vi "SM DEMO.vi"() -> ()   [LabVIEW 2022 SP3, in "StateMachine.lvlib" / "HSE-State-Machine.lvlib"]
doc: "Demonstrates the use of the HSE-State Machine and can be used as a Copy and Paste Template.\n\n____\nHAMPEL SOFTWARE ENGINEERING v2.6.0 (2023-12-19 10:54)"
uses:
  HSE-State-Machine.lvlib
  SM_States.ctl
  SM_Transitions.ctl
  <vilib>/Delacor/Delacor QMH/Libraries/Message Queue_class/Delacor_lib_QMH_Message Queue.lvclass
  <vilib>/Hampel Software Engineering/HSE Logger/hse-logger.lvlib
  Libraries/hse-libraries/Source/hse-dqmh/hse-dqmh.lvlib
panel:
  in  "stop":bool
  in  "Transition":T1=enum."Initialization finished"
  out "SM Exception":errorcluster
  in  "Polling Loop Signal":bool
  out "DEMO State":T2
  # "When HSE-State-Machine.lvlib is copied to another Module\nthan HSE State-Machine-Singleton.lvlib\nright click on the lvlib and select Remove From Library"
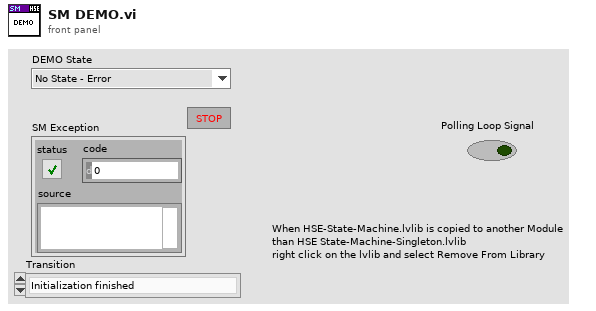
[diagram p1: front panel]
types:
  T1 = typedef "StateMachine.lvlib/HSE-State-Machine.lvlib/SM_Transitions.ctl" = enum16{"No Transition", "Exception", "Reset", "Initialization finished", "Process started", "Trigger detected", "Exit"}
  T2 = typedef "StateMachine.lvlib/HSE-State-Machine.lvlib/SM_States.ctl" = enum16{"No State - Error", "Error - Waiting For Action", "Initialising", "Standing by (idle)", "Waiting for External Trigger", "Polling for Signal Change", "Exiting"}
  T3 = typedef "StateMachine.lvlib/HSE-State-Machine.lvlib/SM Polling Actions--enum.ctl" = enum16{"Check transitions...", "Leave this state!"}
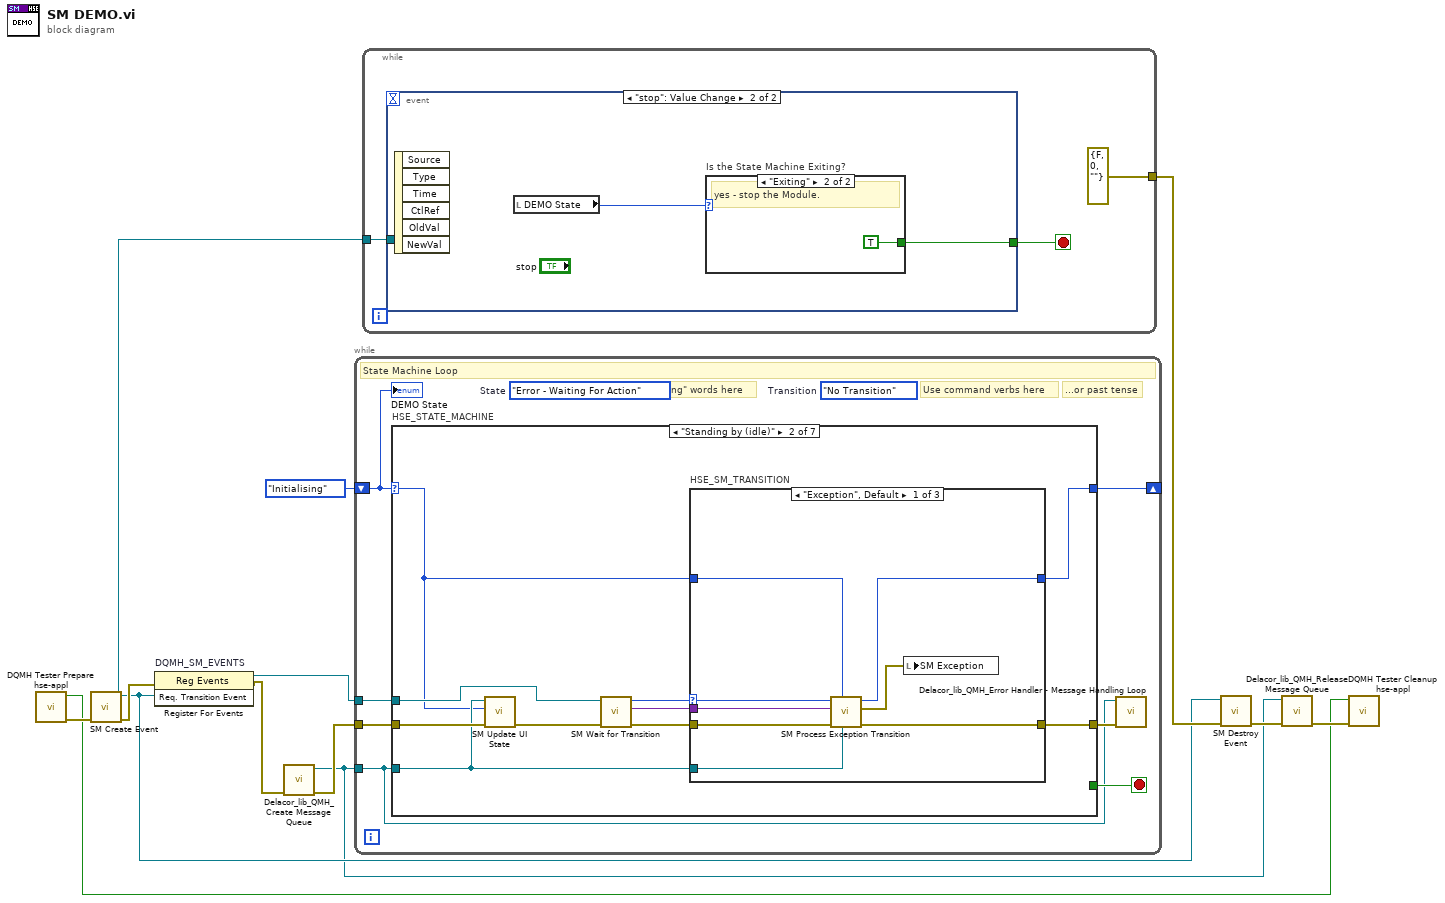
[diagram p0: block diagram]
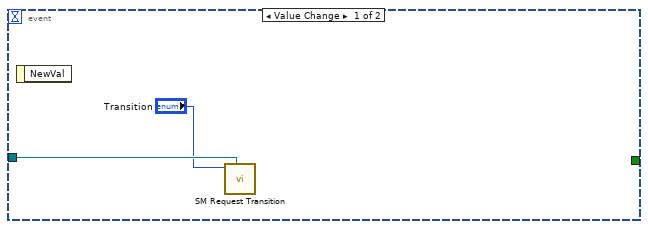
[diagram p2: hidden frame]
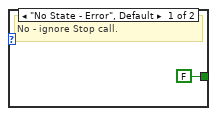
[diagram p3: hidden frame]
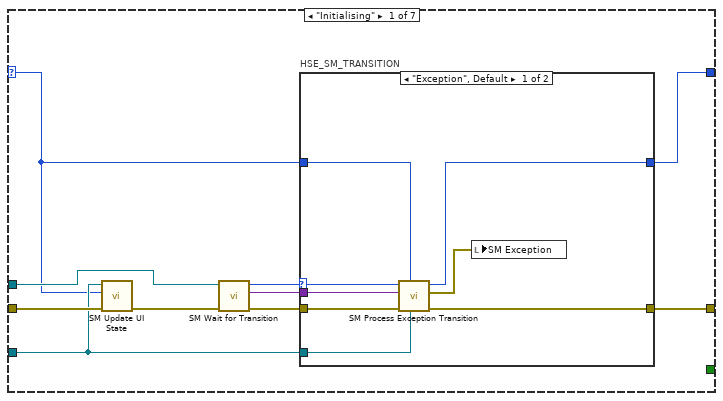
[diagram p4: hidden frame]
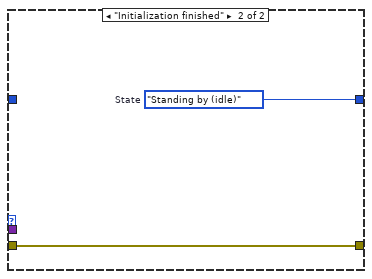
[diagram p5: hidden frame]
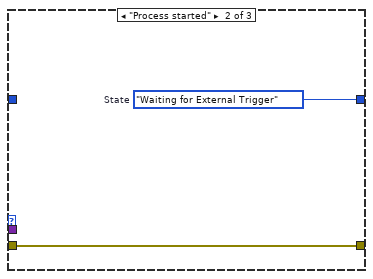
[diagram p6: hidden frame]
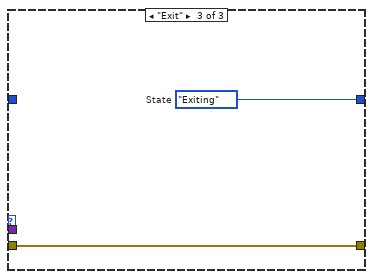
[diagram p7: hidden frame]
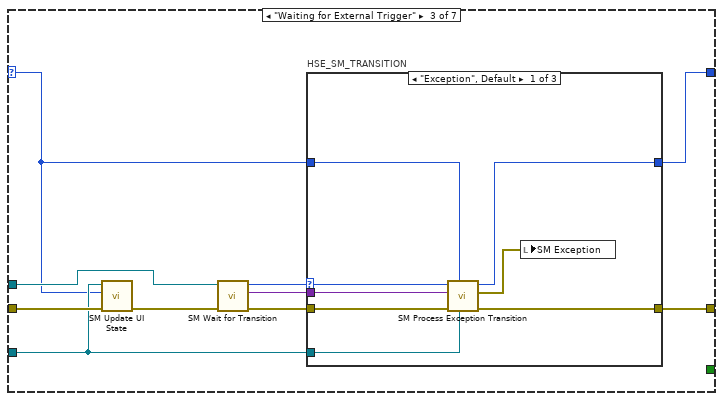
[diagram p8: hidden frame]
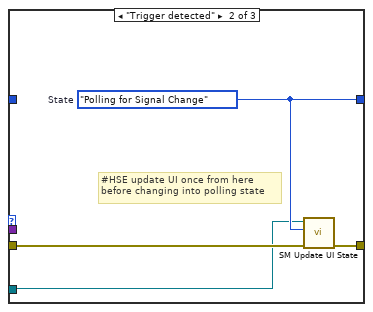
[diagram p9: hidden frame]
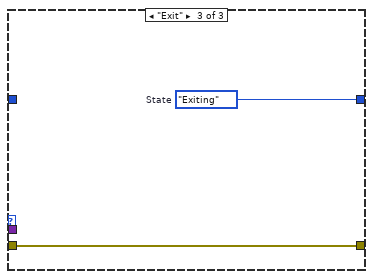
[diagram p10: hidden frame]
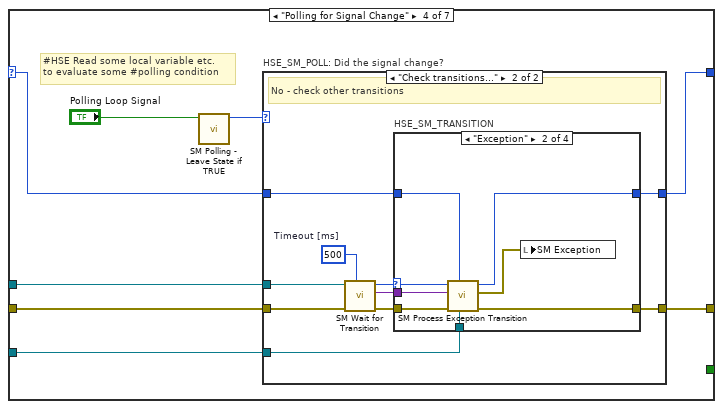
[diagram p11: hidden frame]
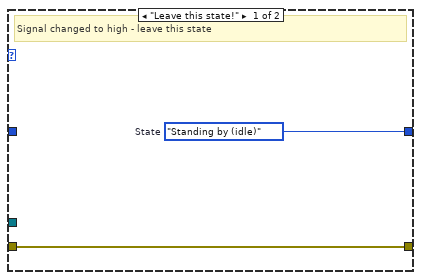
[diagram p12: hidden frame]
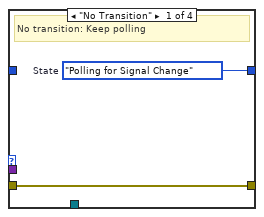
[diagram p13: hidden frame]
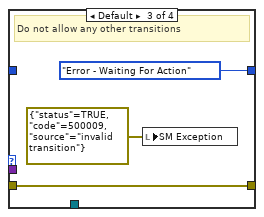
[diagram p14: hidden frame]
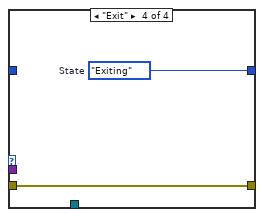
[diagram p15: hidden frame]
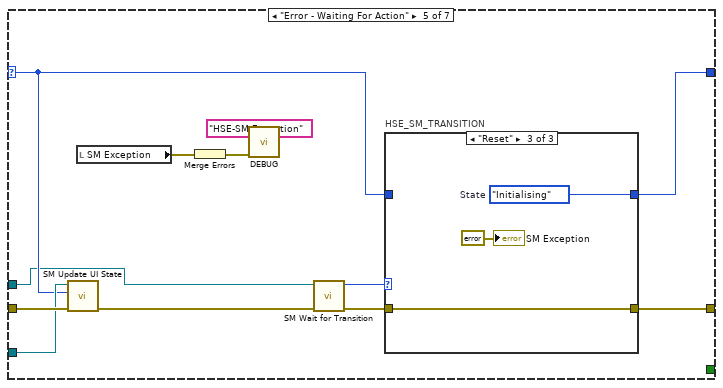
[diagram p16: hidden frame]
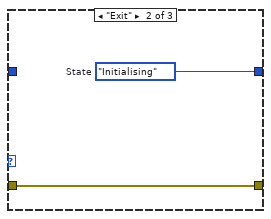
[diagram p18: hidden frame]
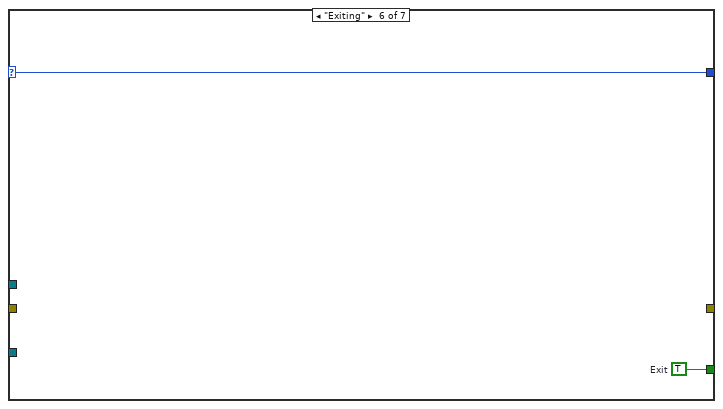
[diagram p19: hidden frame]
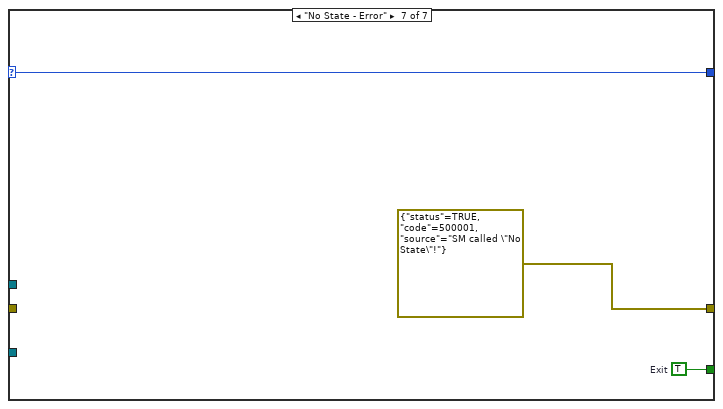
[diagram p20: hidden frame]
diagram:
  n1 = call "DQMH Tester Prepare hse-appl.vi"() -> ("error out"=w2:errorcluster, "Started?"=w1:bool)  [unwired: 8 in, 2 out]
  n2 = call "SM Create Event.vi"("error in (no error)"=w2) -> ("error out"=w10:errorcluster, "Req. Transition Event"=w8:refnum<user-event>)  [unwired: 9 in]
  n3 = register-events "DQMH_SM_EVENTS"(error in=w10, w8) -> (reference out=w9:refnum<event-registration>, error out=w6:errorcluster)  [unwired: 1 in]
  n4 = call <vilib>:"Delacor_lib_QMH_Create Message Queue.vi"("error in"=w6) -> ("error out"=w12:errorcluster, "Message Queue"=w4:refnum<class "Delacor_lib_QMH_Message Queue.lvclass">)  [unwired: 9 in]
  n5 = while {
    shift-right: [w18] -> _
    shift-left: SM_States."Initialising" ("State") -> [w19]
    tunnel: w4 -> [w13]
    tunnel: w9 -> [w15]
    tunnel: w12 -> [w14]
    stop <- w17 stop-if-true
    (unwired) SM_States."Error - Waiting For Action"  # State
    (unwired) SM_Transitions."No Transition"  # Transition
    # "...or past tense"
    # "Use command verbs here"
    # "Use \"-ing\" words here"
    # "State Machine Loop"
    n6 = case "HSE_STATE_MACHINE" shown="\"Standing by (idle)\"" w19 {
      selector: w19 -> [w20 w40 w62 w86 w122 w141 w144]
      tunnel: [w25 w45 w67 w92 w123 w141 w144] -> w18
      tunnel: [_ _ _ _ _ w140 w143] -> w17
      tunnel: w13 -> [w21 w41 w63 w90 w131 _ _]
      tunnel: [w24 w44 w66 w91 w125 _ errorcluster {"status"=TRUE, "code"=500001, "source"="SM called \"No State\"!"} ("error out")] -> w16
      tunnel: w15 -> [w22 w42 w64 w89 w121 _ _]
      tunnel: w14 -> [w29 w49 w71 w93 w132 _ _]
      frame "Initialising" {
        n7 = call "SM Update UI State.vi"("error in (no error)"=w29, "State"=w20, "Message Queue In"=w21) -> ("error out"=w23:errorcluster)  [unwired: 7 in, 1 out]
        n8 = call "SM Wait for Transition.vi"("error in (no error)"=w23, "Event Registration Refnum"=w22) -> ("error out"=w27:errorcluster, "Data"=w26:variant, "Transition"=w28:T1)  [unwired: 7 in]
        n9 = case "HSE_SM_TRANSITION" shown="\"Exception\", Default" w28 {
          selector: w28 -> [w30 _]
          tunnel: w27 -> [w37 w39]
          tunnel: w26 -> [w36 _]
          tunnel: [w32 w38] -> w25
          tunnel: [w35 w39] -> w24
          tunnel: w21 -> [w33 _]
          tunnel: w20 -> [w31 _]
          frame "Exception", Default {
            n10 = call "SM Process Exception Transition.vi"("Message Queue In"=w33, "Exception State"=w31, "error in (no error)"=w37, "Data"=w36, "Exception Transition"=w30) -> ("error out"=w35:errorcluster, "Exception"=w34:errorcluster, "State"=w32:T2)  [unwired: 4 in]
            n11 = local write "SM Exception"(w34) -> ()
          }
          frame "Initialization finished" {
            w38 = SM_States."Standing by (idle)"  # State
          }
        }
      }
      frame "Standing by (idle)" {
        n12 = call "SM Update UI State.vi"("error in (no error)"=w49, "State"=w40, "Message Queue In"=w41) -> ("error out"=w43:errorcluster)  [unwired: 7 in, 1 out]
        n13 = call "SM Wait for Transition.vi"("error in (no error)"=w43, "Event Registration Refnum"=w42) -> ("error out"=w47:errorcluster, "Data"=w46:variant, "Transition"=w48:T1)  [unwired: 7 in]
        n14 = case "HSE_SM_TRANSITION" shown="\"Exception\", Default" w48 {
          selector: w48 -> [w52 _ _]
          tunnel: w47 -> [w57 w59 w61]
          tunnel: w46 -> [w56 _ _]
          tunnel: [w51 w58 w60] -> w45
          tunnel: [w55 w59 w61] -> w44
          tunnel: w41 -> [w53 _ _]
          tunnel: w40 -> [w50 _ _]
          frame "Exception", Default {
            n15 = call "SM Process Exception Transition.vi"("Message Queue In"=w53, "Exception State"=w50, "error in (no error)"=w57, "Data"=w56, "Exception Transition"=w52) -> ("error out"=w55:errorcluster, "Exception"=w54:errorcluster, "State"=w51:T2)  [unwired: 4 in]
            n16 = local write "SM Exception"(w54) -> ()
          }
          frame "Process started" {
            w58 = SM_States."Waiting for External Trigger"  # State
          }
          frame "Exit" {
            w60 = SM_States."Exiting"  # State
          }
        }
      }
      frame "Waiting for External Trigger" {
        n17 = call "SM Update UI State.vi"("error in (no error)"=w71, "State"=w62, "Message Queue In"=w63) -> ("error out"=w65:errorcluster)  [unwired: 7 in, 1 out]
        n18 = call "SM Wait for Transition.vi"("error in (no error)"=w65, "Event Registration Refnum"=w64) -> ("error out"=w69:errorcluster, "Data"=w68:variant, "Transition"=w70:T1)  [unwired: 7 in]
        n19 = case "HSE_SM_TRANSITION" shown="\"Exception\", Default" w70 {
          selector: w70 -> [w72 _ _]
          tunnel: w69 -> [w79 w83 w85]
          tunnel: w68 -> [w78 _ _]
          tunnel: [w74 w81 w84] -> w67
          tunnel: [w77 w82 w85] -> w66
          tunnel: w63 -> [w75 w80 _]
          tunnel: w62 -> [w73 _ _]
          frame "Exception", Default {
            n20 = call "SM Process Exception Transition.vi"("Message Queue In"=w75, "Exception State"=w73, "error in (no error)"=w79, "Data"=w78, "Exception Transition"=w72) -> ("error out"=w77:errorcluster, "Exception"=w76:errorcluster, "State"=w74:T2)  [unwired: 4 in]
            n21 = local write "SM Exception"(w76) -> ()
          }
          frame "Trigger detected" {
            w81 = SM_States."Polling for Signal Change"  # State
            # "#HSE update UI once from here\nbefore changing into polling state"
            n22 = call "SM Update UI State.vi"("error in (no error)"=w83, "State"=w81, "Message Queue In"=w80) -> ("error out"=w82:errorcluster)  [unwired: 7 in, 1 out]
          }
          frame "Exit" {
            w84 = SM_States."Exiting"  # State
          }
        }
      }
      frame "Polling for Signal Change" {
        # "#HSE Read some local variable etc. \nto evaluate some #polling condition"
        n23 = call "SM Polling - Leave State if TRUE.vi"("Boolean Condition"="Polling Loop Signal") -> ("Polling Action"=w88:T3)  [unwired: 10 in]
        n24 = case "HSE_SM_POLL: Did the signal change?" shown="\"Check transitions...\"" w88 {
          tunnel: w93 -> [w94 w105]
          tunnel: [w95 w101] -> w92
          tunnel: [w94 w100] -> w91
          tunnel: w90 -> [_ w99]
          tunnel: w89 -> [_ w98]
          tunnel: w86 -> [_ w96]
          frame "Leave this state!" {
            w95 = SM_States."Standing by (idle)"  # State
            # "Signal changed to high - leave this state"
          }
          frame "Check transitions..." {
            w97 = 500  # Timeout [ms]
            # "No - check other transitions"
            n25 = call "SM Wait for Transition.vi"("Timeout [ms]"=w97, "error in (no error)"=w105, "Event Registration Refnum"=w98) -> ("error out"=w103:errorcluster, "Data"=w102:variant, "Transition"=w104:T1)  [unwired: 6 in]
            n26 = case "HSE_SM_TRANSITION" shown="\"Exception\"" w104 {
              selector: w104 -> [_ w110 _ _]
              tunnel: w103 -> [w106 w115 w117 w120]
              tunnel: w102 -> [_ w114 _ _]
              tunnel: [w107 w109 SM_States."Error - Waiting For Action" ("State") w119] -> w101
              tunnel: [w106 w113 w117 w120] -> w100
              tunnel: w99 -> [_ w111 _ _]
              tunnel: w96 -> [_ w108 _ _]
              frame "No Transition" {
                w107 = SM_States."Polling for Signal Change"  # State
                # "No transition: Keep polling"
              }
              frame "Exception" {
                n27 = call "SM Process Exception Transition.vi"("Message Queue In"=w111, "Exception State"=w108, "error in (no error)"=w115, "Data"=w114, "Exception Transition"=w110) -> ("error out"=w113:errorcluster, "Exception"=w112:errorcluster, "State"=w109:T2)  [unwired: 4 in]
                n28 = local write "SM Exception"(w112) -> ()
              }
              frame Default {
                # "Do not allow any other transitions"
                n29 = local write "SM Exception"(errorcluster {"status"=TRUE, "code"=500009, "source"="invalid transition"} ("SM Exception")) -> ()
              }
              frame "Exit" {
                w119 = SM_States."Exiting"  # State
              }
            }
          }
        }
      }
      frame "Error - Waiting For Action" {
        n30 = call "SM Update UI State.vi"("error in (no error)"=w132, "State"=w122, "Message Queue In"=w131) -> ("error out"=w127:errorcluster)  [unwired: 7 in, 1 out]
        n31 = local read "SM Exception"() -> (w130:errorcluster)
        n32 = Merge Errors(w130) -> (w129:errorcluster)
        n33 = call <vilib>:"DEBUG.vi"("Message"="HSE-SM Exception", "error in"=w129) -> ()  [unwired: 9 in, 1 out]
        n34 = call "SM Wait for Transition.vi"("error in (no error)"=w127, "Event Registration Refnum"=w121) -> ("error out"=w124:errorcluster, "Transition"=w126:T1)  [unwired: 7 in, 1 out]
        n35 = case "HSE_SM_TRANSITION" shown="\"Reset\"" w126 {
          tunnel: [w133 w136 w138] -> w125
          tunnel: w124 -> [w133 w136 w138]
          tunnel: [w134 w135 w139] -> w123
          tunnel: w122 -> [w134 _ _]
          frame Default {
            # "just silently ignore any other transitions"
          }
          frame "Exit" {
            w135 = SM_States."Initialising"  # State
          }
          frame "Reset" {
            w139 = SM_States."Initialising"  # State
            "SM Exception" <- errorcluster {"status"=FALSE, "code"=0, "source"=""} ("SM Exception")
          }
        }
      }
      frame "Exiting" {
        w140 = TRUE  # Exit
      }
      frame "No State - Error" {
        w143 = TRUE  # Exit
      }
    }
    n36 = call-dynamic "Delacor_lib_QMH_Error Handler - Message Handling Loop.vi"("error in"=w16, "Message Queue in"=w13) -> ()  [unwired: 8 in, 2 out]
    "DEMO State" <- w19
  }
  n37 = while {
    tunnel: w8 -> [w147]
    tunnel: [errorcluster {"status"=FALSE, "code"=0, "source"=""} ("error in (no error)")] -> w11
    stop <- w146 stop-if-true
    n38 = event shown="[1] \"stop\": Value Change" {
      selector: _ -> [_ _]
      dyn-events: _ -> [_ _]
      timeout: _ -> [_ _]
      tunnel: w147 -> [w149 _]
      tunnel: [_ w150] -> w146
      event Value Change {
        n39 = event-data() -> ()  [unwired: 1 in, 1 out]
        n40 = call "SM Request Transition.vi"("Req. Transition"=w149, "Transition"="Transition") -> ()  [unwired: 9 in, 1 out]
      }
      event "stop": Value Change {
        n41 = event-data() -> ()  [unwired: 1 in, 6 out]
        n42 = local read "DEMO State"() -> (w151:T2)
        n43 = case "Is the State Machine Exiting?" shown="\"Exiting\"" w151 {
          tunnel: [FALSE TRUE] -> w150
          frame "No State - Error", Default {
            # "No - ignore Stop call."
          }
          frame "Exiting" {
            # "yes - stop the Module."
          }
        }
      }
    }
  }
  n44 = call "SM Destroy Event.vi"("error in (no error)"=w11, "Req. Transition Event"=w8) -> ("error out"=w5:errorcluster)  [unwired: 9 in]
  n45 = call-dynamic "Delacor_lib_QMH_Release Message Queue.vi"("error in"=w5, "Message Queue"=w4) -> ("error out"=w3:errorcluster)  [unwired: 9 in]
  n46 = call "DQMH Tester Cleanup hse-appl.vi"("error in"=w3, "Stop?"=w1) -> ()  [unwired: 9 in, 1 out]
